vi "loop_with_channel.vi"() -> ()   [LabVIEW 2021]
uses:
  <extravilib>/ChannelInstances/Stream-dbl/Read With Abort.vi
  <extravilib>/ChannelInstances/Stream-dbl/Write With Abort.vi
  <extravilib>/ChannelInstances/Stream-dbl/EndpointRead.vi
  <extravilib>/ChannelInstances/Stream-dbl/Endpoint.vi
  <extravilib>/ChannelInstances/Stream-dbl/Instantiate.vi
  <extravilib>/ChannelInstances/Stream-dbl/)Channel.vi
  <resource>/ChannelSupport/_ChannelSupport/WaitIfNeeded.vi
  <extravilib>/ChannelInstances/Stream-dbl.lvlib
panel:
  out "Waveform Chart":dbl(graph)
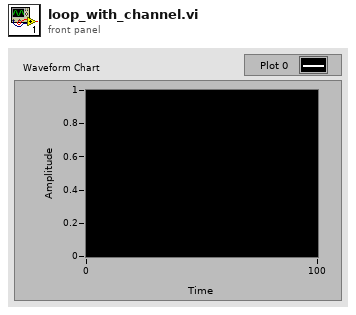
[diagram p1: front panel]
types:
  T1 = typedef "Stream-dbl.lvlib/)Channel.ctl" = refnum<queue>
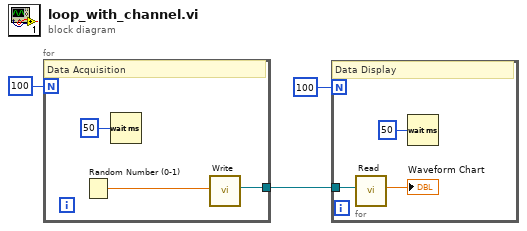
[diagram p0: block diagram]
diagram:
  n1 = for {
    N: 100 -> [_]
    tunnel: [w4] -> w1
    # "Data Acquisition"
    n2 = Random Number (0-1)() -> (number: 0 to 1=w5:dbl)
    n3 = Wait (ms)(milliseconds to wait=u32 50) -> ()  [unwired: 1 out]
    n4 = call <extravilib>:"Write.vi"("element"=w5) -> ("channel"=w4:T1)  [unwired: 8 in, 2 out]
  }
  n5 = for {
    N: 100 -> [_]
    tunnel: w1 -> [w8]
    # "Data Display"
    n6 = call <extravilib>:"Read.vi"("channel"=w8) -> ("element"=→"Waveform Chart":dbl)  [unwired: 6 in, 4 out]
    n7 = Wait (ms)(milliseconds to wait=u32 50) -> ()  [unwired: 1 out]
  }
